vi "Update AO DC.vi"(8 "error in (no error)":errorcluster, 10 "AO.DC (V)":dbl[](array[numeric]), 11 "Generator in":refnum<class "Generator.lvclass">) -> (0 "error out":errorcluster, 3 "Generator out":refnum<class "Generator.lvclass">)   [LabVIEW 2019, in "Generator.lvclass"]
uses:
  Generator/Generator.lvclass
  Generator/Generator.lvclass/Generator.ctl
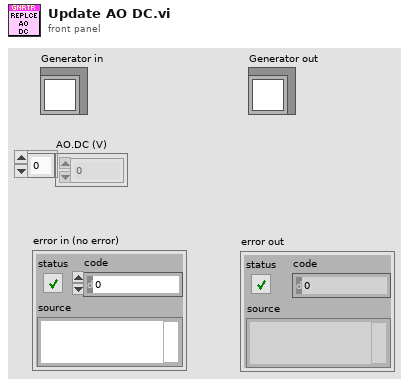
[diagram p1: front panel]
types:
  T1 = typedef "Instrument.Lockin.lvlib/Instrument.DAQ.lvclass/AO.Channel--Cluster--Array.ctl" = T2[]
  T2 = typedef "Instrument.Lockin.lvlib/Instrument.DAQ.lvclass/AO.Channel--Cluster.ctl" = cluster{"Enable?":bool, "Channel":i32, "Amplitude":dbl, "Offset":dbl, "Frequency":dbl, "Phase":dbl, "Function":T3, "Sweeping?":bool, "Limit AC":bool, "Limit DC?":bool}
  T3 = typedef "Instrument.Lockin.lvlib/Instrument.DAQ.lvclass/AO.Channel.Function--Enum.ctl" = enum16{"Sine", "Triangle", "Square"}
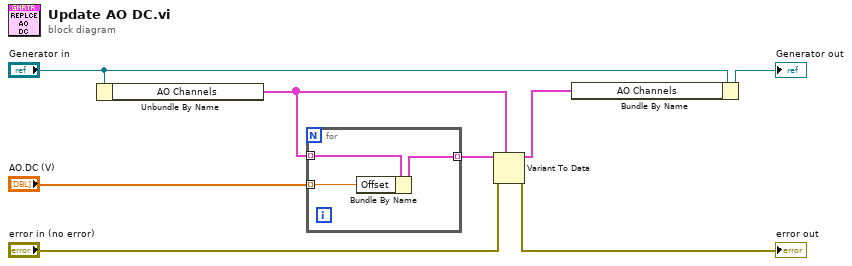
[diagram p0: block diagram]
diagram:
  n1 = Unbundle By Name("Generator in") -> ("AO Channels"=w6:T1)
  n2 = for {
    tunnel: "AO.DC (V)" -> [w11] mode=indexing
    tunnel: w6 -> [w10] mode=indexing
    tunnel: [w9] -> w5 mode=indexing
    n3 = Bundle By Name(cluster=w10, "Offset"=w11) -> (w9:T2)
  }
  n4 = Variant To Data(error in="error in (no error)", type=w6, Variant=w5) -> (data=w4:T1, error out=→"error out":errorcluster)
  n5 = Bundle By Name(cluster="Generator in", "AO Channels"=w4) -> (→"Generator out":refnum<class "Generator.lvclass">)
